vi "check datatype.vi"() -> ()   [LabVIEW 2016]
uses:
  Source/JSON Value/JSON Types.ctl
  Source/JSON Value/JSON Value.lvclass
panel:
  out "matched datatype? 18":bool
  out "matched datatype? 17":bool
  out "matched datatype? 16":bool
  out "matched datatype? 15":bool
  out "matched datatype? 14":bool
  out "matched datatype? 13":bool
  out "matched datatype? 12":bool
  out "matched datatype? 11":bool
  out "matched datatype? 10":bool
  out "matched datatype? 9":bool
  out "matched datatype? 8":bool
  out "matched datatype? 7":bool
  out "matched datatype? 6":bool
  out "matched datatype? 5":bool
  out "matched datatype? 4":bool
  out "matched datatype? 3":bool
  out "matched datatype? 2":bool
  out "matched datatype?":bool
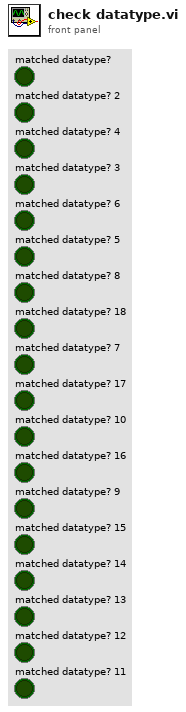
[diagram p1: front panel]
types:
  T1 = typedef "JSON Value.lvclass/JSON Types.ctl" = enum8{"String", "Numeric", "Boolean", "NULL", "Object", "Array"}
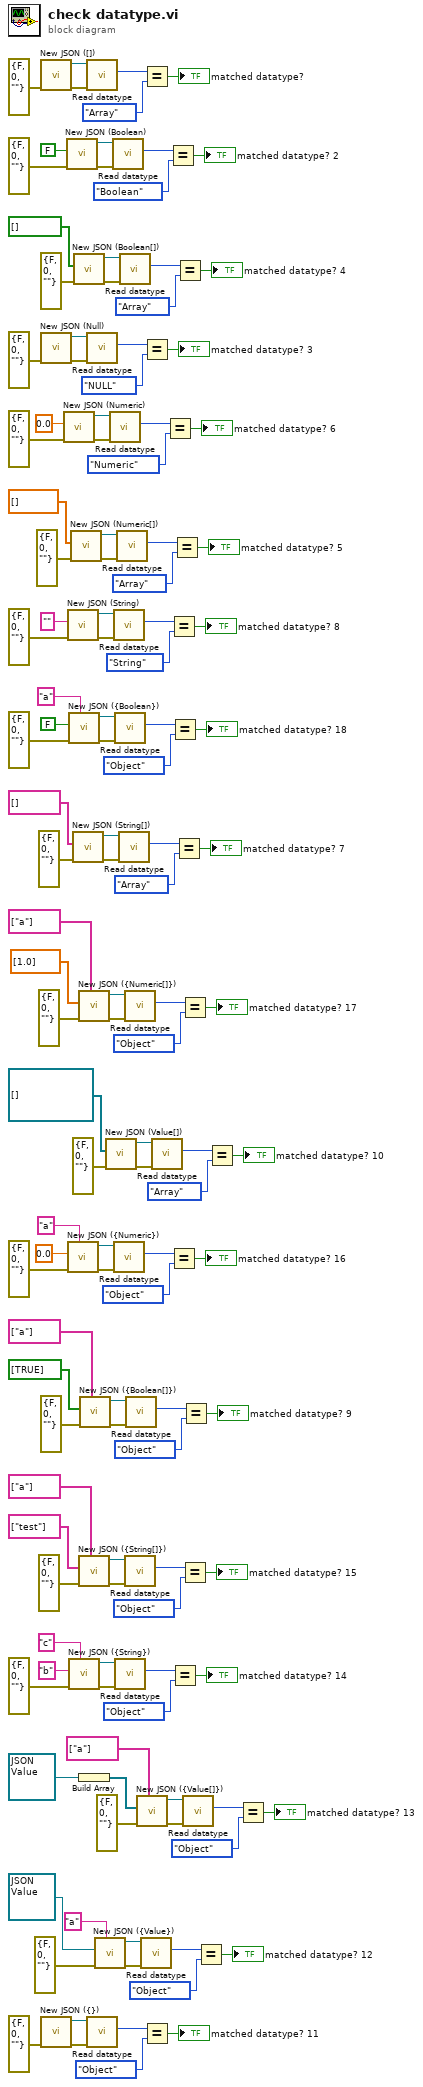
[diagram p0: block diagram]
diagram:
  n1 = call "New JSON ([]).vi"("error in (no error)"=errorcluster {"status"=FALSE, "code"=0, "source"=""}) -> ("error out"=w131:errorcluster, "JSON Value out"=w132:refnum<class "JSON Value.lvclass">)  [unwired: 9 in]
  n2 = call "New JSON (Null).vi"("error in (no error)"=errorcluster {"status"=FALSE, "code"=0, "source"=""}) -> ("error out"=w95:errorcluster, "JSON Value out"=w96:refnum<class "JSON Value.lvclass">)  [unwired: 9 in]
  n3 = call "New JSON ({}).vi"("error in (no error)"=errorcluster {"status"=FALSE, "code"=0, "source"=""}) -> ("error out"=w43:errorcluster, "JSON Value out"=w44:refnum<class "JSON Value.lvclass">)  [unwired: 9 in]
  n4 = call "New JSON (Numeric).vi"("error in (no error)"=errorcluster {"status"=FALSE, "code"=0, "source"=""}, "value"=0.0) -> ("error out"=w93:errorcluster, "JSON Value out"=w94:refnum<class "JSON Value.lvclass">)  [unwired: 8 in]
  n5 = call "New JSON (Boolean).vi"("error in (no error)"=errorcluster {"status"=FALSE, "code"=0, "source"=""}, "value"=FALSE) -> ("error out"=w99:errorcluster, "JSON Value out"=w100:refnum<class "JSON Value.lvclass">)  [unwired: 8 in]
  n6 = call "New JSON (String).vi"("error in (no error)"=errorcluster {"status"=FALSE, "code"=0, "source"=""}, "value"="") -> ("error out"=w89:errorcluster, "JSON Value out"=w90:refnum<class "JSON Value.lvclass">)  [unwired: 8 in]
  n7 = call "New JSON ({Numeric}).vi"("key"="a", "error in (no error)"=errorcluster {"status"=FALSE, "code"=0, "source"=""}, "value"=0.0) -> ("error out"=w53:errorcluster, "JSON Value out"=w54:refnum<class "JSON Value.lvclass">)  [unwired: 7 in]
  n8 = call "New JSON ({Boolean}).vi"("key"="a", "error in (no error)"=errorcluster {"status"=FALSE, "code"=0, "source"=""}, "value"=FALSE) -> ("error out"=w57:errorcluster, "JSON Value out"=w58:refnum<class "JSON Value.lvclass">)  [unwired: 7 in]
  n9 = call "New JSON ({String}).vi"("key"="c", "error in (no error)"=errorcluster {"status"=FALSE, "code"=0, "source"=""}, "value"="b") -> ("error out"=w49:errorcluster, "JSON Value out"=w50:refnum<class "JSON Value.lvclass">)  [unwired: 7 in]
  n10 = call "New JSON (Numeric[]).vi"("error in (no error)"=errorcluster {"status"=FALSE, "code"=0, "source"=""}, "Numeric Array"=dbl[] []) -> ("error out"=w91:errorcluster, "JSON Value out"=w92:refnum<class "JSON Value.lvclass">)  [unwired: 8 in]
  n11 = call "New JSON (String[]).vi"("error in (no error)"=errorcluster {"status"=FALSE, "code"=0, "source"=""}, "String Array"=string[] []) -> ("error out"=w87:errorcluster, "JSON Value out"=w88:refnum<class "JSON Value.lvclass">)  [unwired: 8 in]
  n12 = call "New JSON (Boolean[]).vi"("error in (no error)"=errorcluster {"status"=FALSE, "code"=0, "source"=""}, "Boolean Array"=bool[] []) -> ("error out"=w97:errorcluster, "JSON Value out"=w98:refnum<class "JSON Value.lvclass">)  [unwired: 8 in]
  n13 = call "New JSON ({Numeric[]}).vi"("keys"=string[] ["a"], "error in (no error)"=errorcluster {"status"=FALSE, "code"=0, "source"=""}, "values"=dbl[] [1.0]) -> ("error out"=w55:errorcluster, "JSON Value out"=w56:refnum<class "JSON Value.lvclass">)  [unwired: 7 in]
  n14 = call "New JSON ({String[]}).vi"("keys"=string[] ["a"], "error in (no error)"=errorcluster {"status"=FALSE, "code"=0, "source"=""}, "values"=string[] ["test"]) -> ("error out"=w51:errorcluster, "JSON Value out"=w52:refnum<class "JSON Value.lvclass">)  [unwired: 7 in]
  n15 = Build Array(refnum<class "JSON Value.lvclass"> refnum ("JSON out")) -> (w1:refnum<class "JSON Value.lvclass">[])
  n16 = call "New JSON ({Boolean[]}).vi"("keys"=string[] ["a"], "error in (no error)"=errorcluster {"status"=FALSE, "code"=0, "source"=""}, "values"=bool[] [TRUE]) -> ("error out"=w83:errorcluster, "JSON Value out"=w84:refnum<class "JSON Value.lvclass">)  [unwired: 7 in]
  n17 = call "Read datatype.vi"("error in (no error)"=w131, "JSON Value in"=w132) -> ("datatype"=w130:T1)  [unwired: 7 in, 2 out]
  n18 = call "Read datatype.vi"("error in (no error)"=w95, "JSON Value in"=w96) -> ("datatype"=w124:T1)  [unwired: 7 in, 2 out]
  n19 = call "Read datatype.vi"("error in (no error)"=w43, "JSON Value in"=w44) -> ("datatype"=w82:T1)  [unwired: 7 in, 2 out]
  n20 = call "New JSON ({Value}).vi"("key"="a", "error in (no error)"=errorcluster {"status"=FALSE, "code"=0, "source"=""}, "JSON Value in"=refnum<class "JSON Value.lvclass"> refnum) -> ("error out"=w45:errorcluster, "JSON Value out"=w46:refnum<class "JSON Value.lvclass">)  [unwired: 7 in]
  n21 = call "New JSON (Value[]).vi"("error in (no error)"=errorcluster {"status"=FALSE, "code"=0, "source"=""}, "JSON Datatypes"=refnum<class "JSON Value.lvclass">[] []) -> ("error out"=w85:errorcluster, "JSON Value out"=w86:refnum<class "JSON Value.lvclass">)  [unwired: 8 in]
  n22 = call "Read datatype.vi"("error in (no error)"=w93, "JSON Value in"=w94) -> ("datatype"=w118:T1)  [unwired: 7 in, 2 out]
  n23 = call "Read datatype.vi"("error in (no error)"=w99, "JSON Value in"=w100) -> ("datatype"=w125:T1)  [unwired: 7 in, 2 out]
  n24 = call "Read datatype.vi"("error in (no error)"=w89, "JSON Value in"=w90) -> ("datatype"=w107:T1)  [unwired: 7 in, 2 out]
  n25 = call "Read datatype.vi"("error in (no error)"=w53, "JSON Value in"=w54) -> ("datatype"=w65:T1)  [unwired: 7 in, 2 out]
  n26 = call "Read datatype.vi"("error in (no error)"=w57, "JSON Value in"=w58) -> ("datatype"=w64:T1)  [unwired: 7 in, 2 out]
  n27 = call "Read datatype.vi"("error in (no error)"=w49, "JSON Value in"=w50) -> ("datatype"=w76:T1)  [unwired: 7 in, 2 out]
  n28 = call "Read datatype.vi"("error in (no error)"=w91, "JSON Value in"=w92) -> ("datatype"=w113:T1)  [unwired: 7 in, 2 out]
  n29 = call "Read datatype.vi"("error in (no error)"=w87, "JSON Value in"=w88) -> ("datatype"=w112:T1)  [unwired: 7 in, 2 out]
  n30 = call "Read datatype.vi"("error in (no error)"=w97, "JSON Value in"=w98) -> ("datatype"=w119:T1)  [unwired: 7 in, 2 out]
  n31 = call "Read datatype.vi"("error in (no error)"=w55, "JSON Value in"=w56) -> ("datatype"=w59:T1)  [unwired: 7 in, 2 out]
  n32 = call "Read datatype.vi"("error in (no error)"=w51, "JSON Value in"=w52) -> ("datatype"=w70:T1)  [unwired: 7 in, 2 out]
  n33 = call "Read datatype.vi"("error in (no error)"=w83, "JSON Value in"=w84) -> ("datatype"=w101:T1)  [unwired: 7 in, 2 out]
  n34 = call "New JSON ({Value[]}).vi"("keys"=string[] ["a"], "error in (no error)"=errorcluster {"status"=FALSE, "code"=0, "source"=""}, "values"=w1) -> ("error out"=w47:errorcluster, "JSON Value out"=w48:refnum<class "JSON Value.lvclass">)  [unwired: 7 in]
  n35 = call "Read datatype.vi"("error in (no error)"=w45, "JSON Value in"=w46) -> ("datatype"=w77:T1)  [unwired: 7 in, 2 out]
  n36 = Equal?(x=w130, y=JSON_Types."Array") -> (x = y?=→"matched datatype?":bool)
  n37 = Equal?(x=w124, y=JSON_Types."NULL") -> (x = y?=→"matched datatype? 3":bool)
  n38 = Equal?(x=w82, y=JSON_Types."Object") -> (x = y?=→"matched datatype? 11":bool)
  n39 = call "Read datatype.vi"("error in (no error)"=w85, "JSON Value in"=w86) -> ("datatype"=w106:T1)  [unwired: 7 in, 2 out]
  n40 = Equal?(x=w118, y=JSON_Types."Numeric") -> (x = y?=→"matched datatype? 6":bool)
  n41 = Equal?(x=w125, y=JSON_Types."Boolean") -> (x = y?=→"matched datatype? 2":bool)
  n42 = Equal?(x=w107, y=JSON_Types."String") -> (x = y?=→"matched datatype? 8":bool)
  n43 = Equal?(x=w65, y=JSON_Types."Object") -> (x = y?=→"matched datatype? 16":bool)
  n44 = Equal?(x=w64, y=JSON_Types."Object") -> (x = y?=→"matched datatype? 18":bool)
  n45 = Equal?(x=w76, y=JSON_Types."Object") -> (x = y?=→"matched datatype? 14":bool)
  n46 = Equal?(x=w113, y=JSON_Types."Array") -> (x = y?=→"matched datatype? 5":bool)
  n47 = Equal?(x=w112, y=JSON_Types."Array") -> (x = y?=→"matched datatype? 7":bool)
  n48 = Equal?(x=w119, y=JSON_Types."Array") -> (x = y?=→"matched datatype? 4":bool)
  n49 = Equal?(x=w59, y=JSON_Types."Object") -> (x = y?=→"matched datatype? 17":bool)
  n50 = Equal?(x=w70, y=JSON_Types."Object") -> (x = y?=→"matched datatype? 15":bool)
  n51 = Equal?(x=w101, y=JSON_Types."Object") -> (x = y?=→"matched datatype? 9":bool)
  n52 = call "Read datatype.vi"("error in (no error)"=w47, "JSON Value in"=w48) -> ("datatype"=w71:T1)  [unwired: 7 in, 2 out]
  n53 = Equal?(x=w77, y=JSON_Types."Object") -> (x = y?=→"matched datatype? 12":bool)
  n54 = Equal?(x=w106, y=JSON_Types."Array") -> (x = y?=→"matched datatype? 10":bool)
  n55 = Equal?(x=w71, y=JSON_Types."Object") -> (x = y?=→"matched datatype? 13":bool)
